vi "Find COM port update.vi"() -> (1 "Comm Successful":bool, 2 "VISA resource name out":refnum<visa-resource-name>)   [LabVIEW 2017]
uses:
  <vilib>/Instr/_visa.llb/VISA Configure Serial Port (Instr).vi
panel:
  out "find list":string[](array[string])
  out "element":string
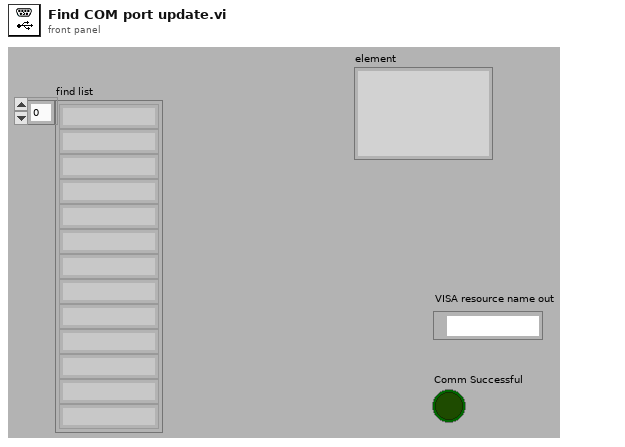
[diagram p1: front panel]
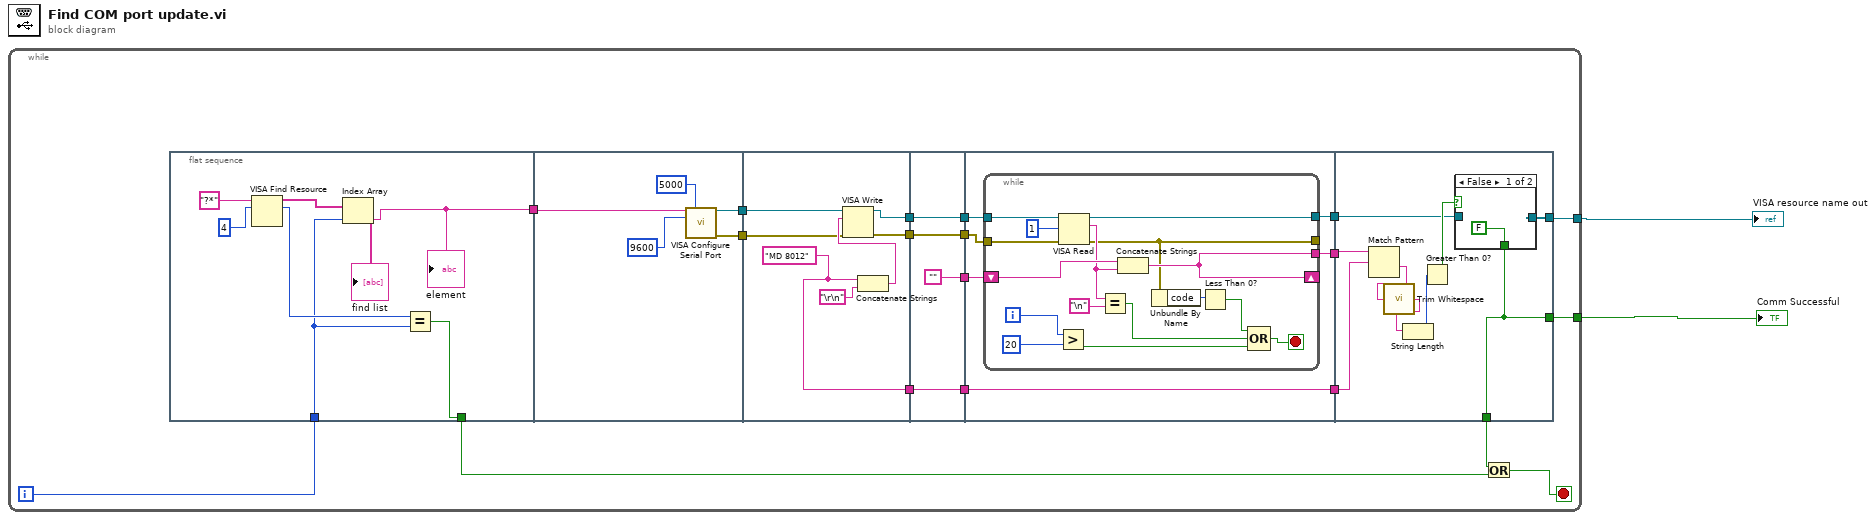
[diagram p0: block diagram]
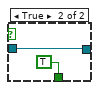
[diagram p2: hidden frame]
diagram:
  n1 = while {
    tunnel: [w21] -> w2
    tunnel: [w20] -> w1
    i -> [w6]
    stop <- w5 stop-if-true
    n2 = flat-sequence {
      tunnel: [w22] -> w7
      tunnel: w6 -> [w24]
      tunnel: [w25] -> _
      tunnel: [w25] -> w3
      tunnel: [w30] -> w19
      tunnel: [w31] -> w18
      tunnel: w7 -> [w29]
      tunnel: [w38] -> w17
      tunnel: [w37] -> w16
      tunnel: [w36] -> w15
      tunnel: w19 -> [w35]
      tunnel: w18 -> [w34]
      tunnel: [w44] -> w14
      tunnel: w17 -> [w44]
      tunnel: [w43] -> w13
      tunnel: w16 -> [w43]
      tunnel: [""] -> w12
      tunnel: [w41] -> w11
      tunnel: w15 -> [w41]
      tunnel: w14 -> [w50]
      tunnel: w13 -> [w49]
      tunnel: w12 -> [w47]
      tunnel: [w48] -> w10
      tunnel: [w46] -> w9
      tunnel: w11 -> [w46]
      tunnel: [w45] -> w8
      tunnel: w10 -> [w71]
      tunnel: w9 -> [w72]
      tunnel: w8 -> [w74]
      tunnel: [w73] -> w21
      tunnel: [w67] -> w20
      tunnel: [w67] -> w4
      frame #0 {
        n3 = VISA Find Resource(10:4, 11:"?*") -> (2:w26:u32, 3:w23:string[])  [unwired: 1 in, 1 out]
        "find list" <- w23
        n4 = Index Array(array=w23, index=w24) -> (element=w22:string)
        "element" <- w22
        n5 = Equal?(x=w26, y=w24) -> (x = y?=w25:bool)
      }
      frame #1 {
        n6 = call-poly "VISA Configure Serial Port"("VISA resource name"=w29, "timeout (10sec)"=u32 5000 ("baud rate (9600)"), "baud rate (9600)"=u32 9600) -> ("VISA resource name out"=w30:refnum<visa-resource-name>, "error out"=w31:errorcluster)  [unwired: 11 in]
      }
      frame #2 {
        w36 = "MD 8012"
        n7 = Concatenate Strings(w36, "\r\n") -> (w39:string)
        n8 = VISA Write(VISA resource name=w35, write buffer=w39, error in (no error)=w34) -> (VISA resource name out=w38:refnum<visa-resource-name>, error out=w37:errorcluster)  [unwired: 1 out]
      }
      frame #3 {
      }
      frame #4 {
        n9 = while {
          tunnel: [w66] -> w45
          tunnel: [w53] -> _
          tunnel: [w63] -> w48
          shift-right: [w63] -> _
          shift-left: w47 -> [w64]
          tunnel: w50 -> [w61]
          tunnel: w49 -> [w60]
          i -> [w59]
          stop <- w57 stop-if-true
          n10 = Greater?(x=w59, y=20) -> (0:w56:bool)
          n11 = VISA Read(VISA resource name=w61, byte count=1, error in (no error)=w60) -> (VISA resource name out=w66:refnum<visa-resource-name>, read buffer=w62:string, error out=w53:errorcluster)  [unwired: 1 out]
          n12 = Equal?(x=w62, y="\n") -> (x = y?=w54:bool)
          n13 = Concatenate Strings(w64, w62) -> (w63:string)
          n14 = Unbundle By Name(w53) -> ("code"=w52:i32)
          n15 = Less Than 0?(x=w52) -> (x < 0?=w51:bool)
          n16 = Compound Arithmetic op=OR(w51, w54, w56) -> (w57:bool)
        }
      }
      frame #5 {
        n17 = Match Pattern(string=w71, regular expression=w72) -> (after substring=w68:string)  [unwired: 1 in, 3 out]
        n18 = call <vilib>:"Trim Whitespace.vi"("string"=w68) -> ("trimmed string"=w69:string)  [unwired: 1 in]
        n19 = String Length(string=w69) -> (length=w70:i32)
        n20 = Greater Than 0?(x=w70) -> (x > 0?=w75:bool)
        n21 = case shown="False" w75 {
          tunnel: [_ w78] -> w73
          tunnel: w74 -> [_ w78]
          tunnel: [FALSE TRUE] -> w67
          frame False {
          }
          frame True {
          }
        }
      }
    }
    n22 = Or(x=w4, y=w3) -> (x .or. y?=w5:bool)
  }
  "VISA resource name out" <- w2
  "Comm Successful" <- w1
